vi "9217_Initialize.vi"(8 "error in (no error)":errorcluster, 9 "Slot Settings":T1, 11 "9217 in":refnum<class "9217.lvclass">) -> (0 "error out":errorcluster, 3 "9217 out":refnum<class "9217.lvclass">)   [LabVIEW 2020, in "Modules.lvlib" / "9217.lvclass"]
uses:
  9217.lvclass
  RSI Module/Slot Settings.ctl
  C:/Users/nitest/Desktop/Git 2020/niveristand-scan-engine-module-libraries/Source/RSI Module/RSI Module.lvclass
  RSI Module/Channels.ctl
  RSI Module/Channel Type.ctl
  RSI Module/Module Models.ctl
  9217.lvclass/9217.ctl
  RSI Module/RSI Module.lvclass
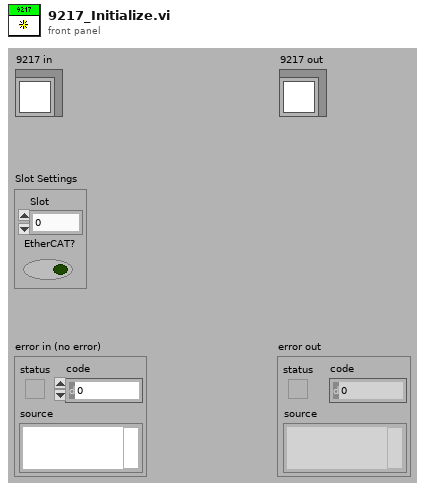
[diagram p1: front panel]
types:
  T1 = typedef "Modules.lvlib/RSI Module.lvclass/Slot Settings.ctl" = cluster{"Slot":u32, "EtherCAT?":bool}
  T2 = typedef "Modules.lvlib/RSI Module.lvclass/Module Models.ctl" = enum16{"Empty", "NI 9201", "NI 9203", "NI 9205", "NI 9206", "NI 9207", "NI 9208", "NI 9209", "NI 9210", "NI 9211", "NI 9212", "NI 9213", "NI 9214", "NI 9215", "NI 9216", "NI 9217", "NI 9219", "NI 9220", "NI 9221", "NI 9222", "NI 9223", "NI 9224", "NI 9225", "NI 9226", "NI 9227", "NI 9228", "NI 9229", "NI 9233", "NI 9234", "NI 9235", "NI 9236", "NI 9237", "NI 9239", "NI 9242", "NI 9244", "NI 9253", "NI 9263", "NI 9264", "NI 9265", "NI 9266", "NI 9269", "NI 9344", "NI 9350", "NI 9375", "NI 9401", "NI 9402", "NI 9403", "NI 9411", "NI 9421", "NI 9422", "NI 9423", "NI 9425", "NI 9426", "NI 9435", "NI 9436", "NI 9437", "NI 9472", "NI 9474", "NI 9475", "NI 9476", "NI 9477", "NI 9478", "NI 9481", "NI 9482", "NI 9485"}
  T3 = cluster{"Ohm degree range":u32, "RTD type":u32, "RTD user-defined A constant":dbl, "RTD user-defined B constant":dbl, "RTD user-defined C constant":dbl, "RTD user-defined Ro constant":dbl}
  T4 = typedef "Modules.lvlib/RSI Module.lvclass/Channels.ctl" = cluster{"# Input Channels":i32, "# Output Channels":i32, "Channel Type":T5, "Units":string}
  T5 = typedef "Modules.lvlib/RSI Module.lvclass/Channel Type.ctl" = enum16{"Analog", "Digital"}
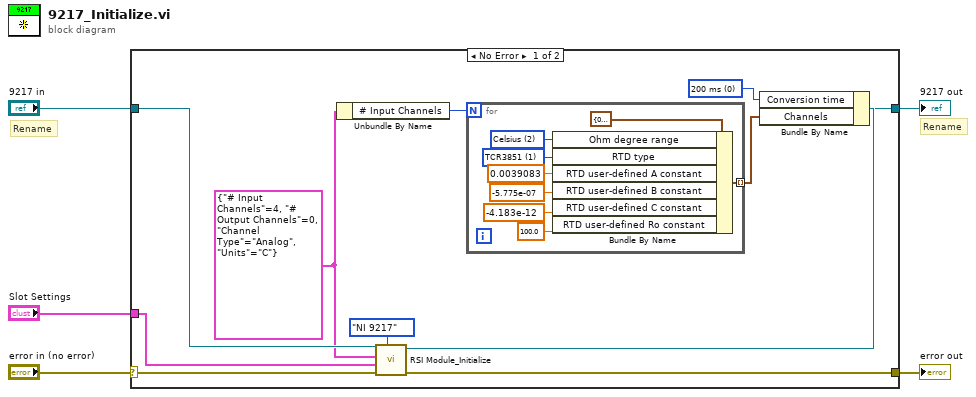
[diagram p0: block diagram]
diagram:
  # "Rename"
  # "Rename"
  n1 = case shown="No Error" "error in (no error)" {
    selector: "error in (no error)" -> [w14 w26]
    tunnel: [w13 w26] -> w4
    tunnel: [w11 w25] -> w2
    tunnel: "9217 in" -> [w16 w25]
    tunnel: "Slot Settings" -> [w15 _]
    frame No Error {
      w9 = u32 0 items=["200 ms", "2.5 ms"] ("Conversion time")
      w8 = T4 {"# Input Channels"=4, "# Output Channels"=0, "Channel Type"=enum."Analog", "Units"="C"} ("Channels")
      n2 = Unbundle By Name(w8) -> ("# Input Channels"=w7:i32)
      n3 = call "RSI Module_Initialize.vi"("Module Model"=Module_Models."NI 9217", "error in (no error)"=w14, "Slot Settings"=w15, "Channels"=w8, "RSI Module in"=w16) -> ("error out"=w13:errorcluster, "RSI Module out"=w12:refnum<class "9217.lvclass">)  [unwired: 5 in]
      n4 = for {
        N: w7 -> [_]
        tunnel: [w23] -> w6 mode=indexing
        w21 = u32 1 items=["User Defined", "TCR3851", "TCR3750", "TCR3916", "TCR3920", "TCR3911", "TCR3928"] ("RTD type")
        w22 = u32 2 items=["Ohms", "Kelvin", "Celsius", "Fahrenheit", "Rankine"] ("Ohm degree range")
        n5 = Bundle By Name(cluster=T3 {"Ohm degree range"=0, "RTD type"=0, "RTD user-defined A constant"=0.0, "RTD user-defined B constant"=0.0, "RTD user-defined C constant"=0.0, "RTD user-defined Ro constant"=0.0} ("Channel"), "Ohm degree range"=w22, "RTD type"=w21, "RTD user-defined A constant"=0.0039083, "RTD user-defined B constant"=-5.775e-07, "RTD user-defined C constant"=-4.183e-12, "RTD user-defined Ro constant"=100.0) -> (w23:T3)
      }
      n6 = Bundle By Name(cluster=w12, "Conversion time"=w9, "Channels"=w6) -> (w11:refnum<class "9217.lvclass">)
    }
    frame Error {
    }
  }
  "error out" <- w4
  "9217 out" <- w2
